vi "Nudge Position Up.vi"(8 "error in (no error)":errorcluster, 11 "MulticolumnListbox in":refnum<vi>) -> (0 "error out":errorcluster)   [LabVIEW 2020, in "ListboxExtensions.lvlib"]
doc: "向上移动位置"
uses:
  ListboxExtensions.lvlib
  <vilib>/Utility/miscctls.llb/LVRowAndColumnUnsignedTypeDef.ctl
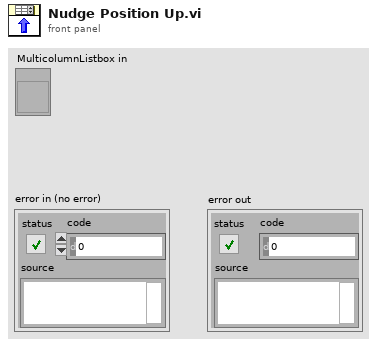
[diagram p1: front panel]
types:
  T1 = typedef "LVRowAndColumnUnsignedTypeDef.ctl" = cluster{"Row":u32, "Column":u32}
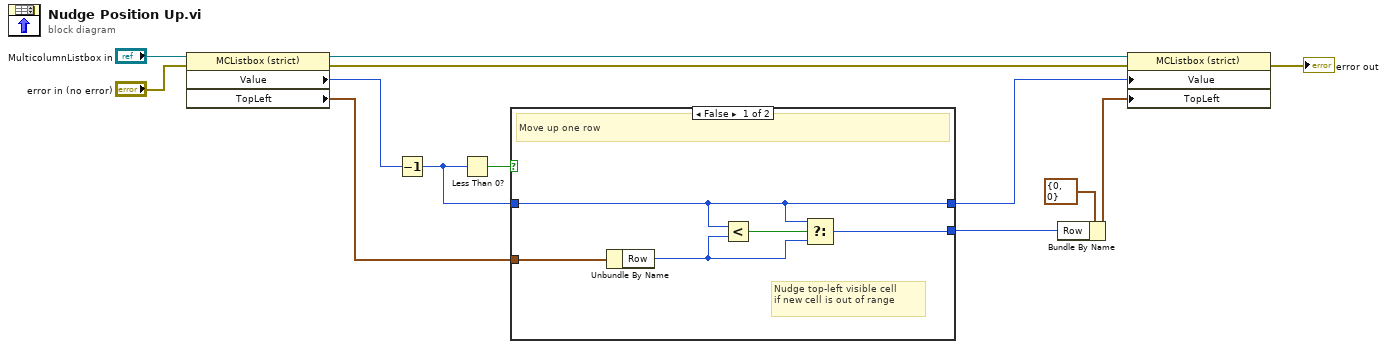
[diagram p0: block diagram]
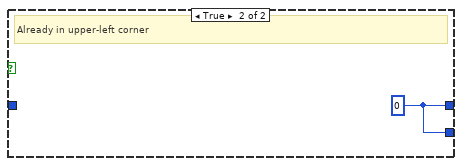
[diagram p2: hidden frame]
diagram:
  n1 = property class="MCListbox (strict)"(reference="MulticolumnListbox in", error in="error in (no error)") -> (reference out=w7:refnum<vi>, error out=w6:errorcluster, "Value"=w5:i32, "TopLeft"=w12:T1)
  n2 = Decrement(x=w5) -> (x-1=w13:i32)
  n3 = Less Than 0?(x=w13) -> (x < 0?=w9:bool)
  n4 = case shown="False" w9 {
    tunnel: [w16 w19] -> w10
    tunnel: [w14 w19] -> w11
    tunnel: w12 -> [w18 _]
    tunnel: w13 -> [w16 _]
    frame False {
      # "Nudge top-left visible cell\nif new cell is out of range"
      # "Move up one row"
      n5 = Unbundle By Name(w18) -> ("Row"=w15:u32)
      n6 = Less?(x=w16, y=w15) -> (x < y?=w17:bool)
      n7 = Select(t=w16, s=w17, f=w15) -> (s? t:f=w14:u32)
    }
    frame True {
      w19 = 0 ("lower limit")
      # "Already in upper-left corner"
    }
  }
  n8 = Bundle By Name(cluster=T1 {"Row"=0, "Column"=0} ("Top Left Visible Cell"), "Row"=w11) -> (w2:T1)
  n9 = property class="MCListbox (strict)"(reference=w7, error in=w6, "Value"=w10, "TopLeft"=w2) -> (error out=→"error out":errorcluster)  [unwired: 1 out]
